vi "Create LSTM Cell.vi"() -> ()   [LabVIEW 2020]
panel:
  in  "weight path":path
  in  "name":string
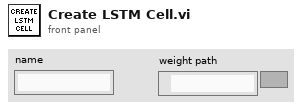
[diagram p1: front panel]
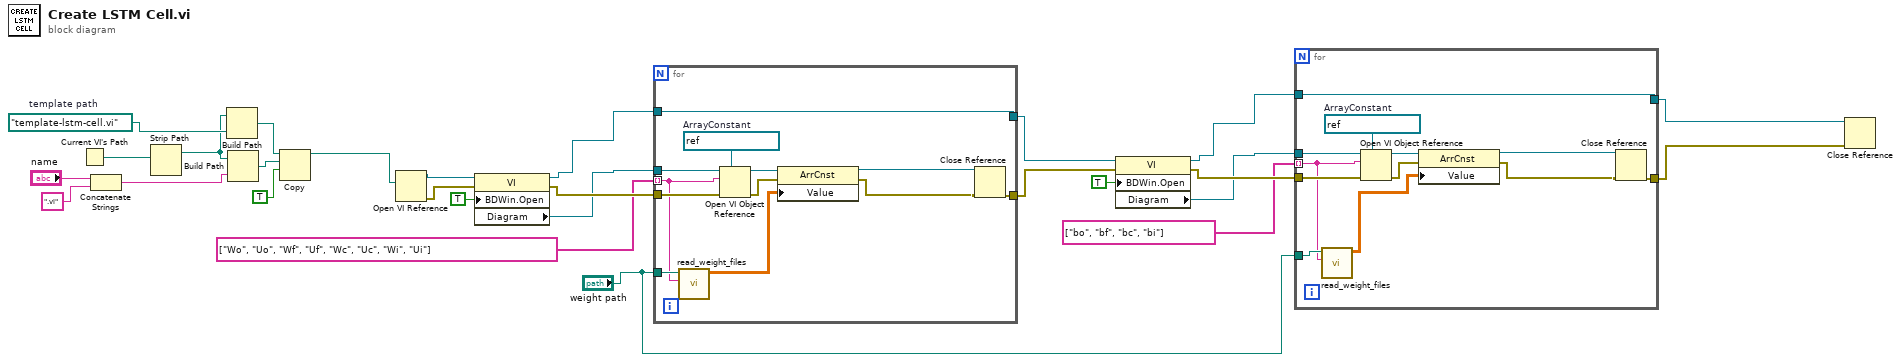
[diagram p0: block diagram]
diagram:
  w6 = path "template-lstm-cell.vi"  # template path
  n1 = Current VI's Path() -> (path=w5:path)
  n2 = Concatenate Strings("name", ".vi") -> (w7:string)
  n3 = Strip Path(path=w5) -> (stripped path=w4:path)  [unwired: 1 out]
  n4 = Build Path(base path=w4, name or relative path=w6) -> (appended path=w2:path)
  n5 = Build Path(base path=w4, name or relative path=w7) -> (appended path=w1:path)
  n6 = Copy(9:TRUE, 10:w1, 11:w2) -> (3:w22:path)  [unwired: 2 in, 2 out]
  n7 = Open VI Reference(vi path=w22) -> (vi reference=w24:refnum<vi>, error out=w23:errorcluster)  [unwired: 5 in]
  n8 = property class="VI"(reference=w24, error in=w23, "BDWin.Open"=TRUE) -> (reference out=w20:refnum<vi>, error out=w26:errorcluster, "Diagram"=w21:refnum<vi>)
  n9 = for {
    tunnel: w26 -> [w39]
    tunnel: w21 -> [w38]
    tunnel: string[] ["Wo", "Uo", "Wf", "Uf", "Wc", "Uc", "Wi", "Ui"] -> [w29] mode=indexing
    tunnel: [w33] -> w13
    tunnel: "weight path" -> [w30]
    tunnel: [w34] -> w14
    tunnel: w20 -> [w34]
    w37 = refnum<vi> refnum  # ArrayConstant
    n10 = call "read_weight_files.vi"("weight file name"=w29, "weights path"=w30) -> ("all rows"=w28:dbl[][])  [unwired: 9 in]
    n11 = Open VI Object Reference(7:w37, 8:w39, 10:w29, 11:w38) -> (0:w35:errorcluster, 3:w36:refnum<vi>)
    n12 = property class="ArrCnst"(reference=w36, error in=w35, "Value"=w28) -> (reference out=w32:refnum<vi>, error out=w31:errorcluster)
    n13 = Close Reference(reference=w32, error in (no error)=w31) -> (error out=w33:errorcluster)
  }
  n14 = property class="VI"(reference=w14, error in=w13, "BDWin.Open"=TRUE) -> (reference out=w15:refnum<vi>, error out=w17:errorcluster, "Diagram"=w16:refnum<vi>)
  n15 = for {
    tunnel: w17 -> [w51]
    tunnel: w16 -> [w50]
    tunnel: string[] ["bo", "bf", "bc", "bi"] -> [w41] mode=indexing
    tunnel: [w45] -> w10
    tunnel: "weight path" -> [w42]
    tunnel: [w46] -> w11
    tunnel: w15 -> [w46]
    w49 = refnum<vi> refnum  # ArrayConstant
    n16 = call "read_weight_files.vi"("weight file name"=w41, "weights path"=w42) -> ("all rows"=w40:dbl[][])  [unwired: 9 in]
    n17 = Open VI Object Reference(7:w49, 8:w51, 10:w41, 11:w50) -> (0:w47:errorcluster, 3:w48:refnum<vi>)
    n18 = property class="ArrCnst"(reference=w48, error in=w47, "Value"=w40) -> (reference out=w44:refnum<vi>, error out=w43:errorcluster)
    n19 = Close Reference(reference=w44, error in (no error)=w43) -> (error out=w45:errorcluster)
  }
  n20 = Close Reference(reference=w11, error in (no error)=w10) -> ()  [unwired: 1 out]
